vi "Initialize SLSC Switch Custom Device.vi"(8 "error in":errorcluster, 11 "slsc switch custom device in":T1 format="%.0x") -> (0 "error out":errorcluster, 2 "endpoint configuration section":T1 format="%.0x", 3 "slsc switch custom device out":T1 format="%.0x")   [LabVIEW 2020, in "SLSC Switch Scripting.lvlib"]
uses:
  SLSC Switch Scripting.lvlib
  <vilib>/NI VeriStand/Custom Device API/Custom Device Item Ref.ctl
  Properties/SLSC Switch All Properties.ctl
  SLSC Scripting Constants.vi
  Shared/Constants.vi
  <vilib>/NI VeriStand/Custom Device API/Custom Device API.lvlib
  Dependencies.llb/SLSC Switch Shared.lvlib
  Routing and Faulting/Routing and Faulting Hardware API/Routing and Faulting Hardware API.lvlib
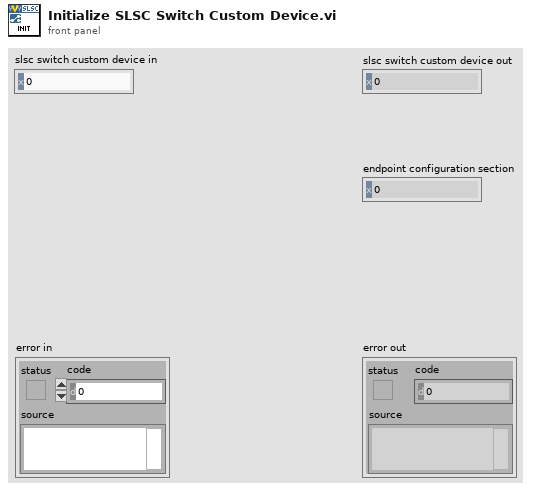
[diagram p1: front panel]
types:
  T1 = typedef "Custom Device API.lvlib/Custom Device Item Ref.ctl" = u64
  T2 = typedef "SLSC Switch Scripting.lvlib/SLSC Switch All Properties.ctl" = cluster{"Product Name":string, "Topology":string, "Switches JSON":string, "Description":string, "Reservation Group":string}
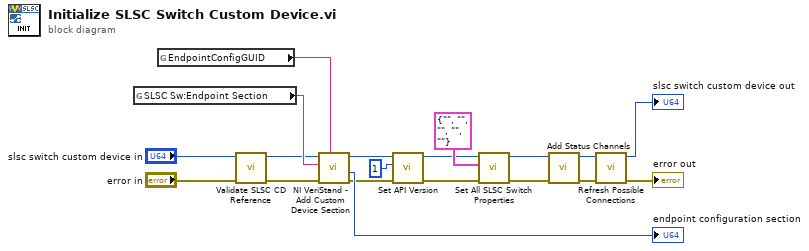
[diagram p0: block diagram]
diagram:
  n1 = global read "SLSC Scripting Constants.vi" "SLSC Sw:Endpoint Section"() -> (w18:string)
  n2 = global read "Constants.vi" "EndpointConfigGUID"() -> (w15:string)
  n3 = call "Validate SLSC CD Reference.vi"("error in"="error in", "slsc switch custom device in"="slsc switch custom device in") -> ("error out"=w7:errorcluster, "slsc switch custom device out"=w5:T1)  [unwired: 8 in]
  n4 = call <vilib>:"NI VeriStand - Add Custom Device Section.vi"("GUID (Default Section)"=w15, "error in (no error)"=w7, "Section Name"=w18, "Parent Ref in"=w5) -> ("error out"=w11:errorcluster, "Section Ptr"=→"endpoint configuration section":T1, "Parent Ref out"=w12:T1)  [unwired: 4 in, 1 out]
  n5 = call "Set API Version.vi"("error in (no error)"=w11, "API version"=u32 1, "Hardware Ref in"=w12) -> ("error out"=w10:errorcluster, "Hardware Ref out"=w9:T1)  [unwired: 7 in]
  n6 = call "Set All SLSC Switch Properties.vi"("error in"=w10, "properties"=T2 {"Product Name"="", "Topology"="", "Switches JSON"="", "Description"="", "Reservation Group"=""} ("SLSC Switch All Properties"), "slsc switch custom device in"=w9) -> ("error out"=w14:errorcluster, "slsc switch custom device out"=w13:T1)  [unwired: 7 in]
  n7 = call "Add Status Channels.vi"("error in"=w14, "slsc switch custom device in"=w13) -> ("error out"=w4:errorcluster, "slsc switch custom device out"=w3:T1)  [unwired: 8 in]
  n8 = call "Refresh Possible Connections.vi"("error in"=w4, "slsc switch custom device in"=w3) -> ("error out"=→"error out":errorcluster, "slsc switch custom device out"=→"slsc switch custom device out":T1)  [unwired: 8 in]
